vi "main.vi"() -> ()   [LabVIEW 2023]
uses:
  Lens Driver (20.06.2016)/03 Type Def & Global/Calibration.ctl
  <vilib>/Instr/_visa.llb/VISA Configure Serial Port (Instr).vi
panel:
  in  "Slide":dbl(slide) scale=0.0..10.0
  out "TA (°C)":dbl
  in  "Read Temperature":bool caption="Send Command"
  out "Command to Port":string
  in  "Current Ch A (mA)":dbl
  out "Data":string
  out "OK":bool
  out "Calibration 2":T1 {"Max Current A" format="%#_g mA"; "Max Current B" format="%#_g mA"; "UCL A" format="%#_g mA"; "LCL A" format="%#_g mA"; "UCL B" format="%#_g mA"; "LCL B" format="%#_g mA"}
  out "VISA resource name out":string
  in  "stop":bool
  in  "Send command":bool caption="Send Command"
  out "ID":u16
  out "error out":errorcluster
  in  "Calibration":T1={"Max Current A"=293.0, "Max Current B"=293.0, "UCL A"=300.0, "UCL B"=300.0, "LCL A"=0.0, "LCL B"=0.0} {"Max Current A" format="%#_g mA"; "Max Current B" format="%#_g mA"; "UCL A" format="%#_g mA"; "LCL A" format="%#_g mA"; "UCL B" format="%#_g mA"; "LCL B" format="%#_g mA"}
  in  "error in (no error)":errorcluster
  in  "VISA resource name":string="COM5"
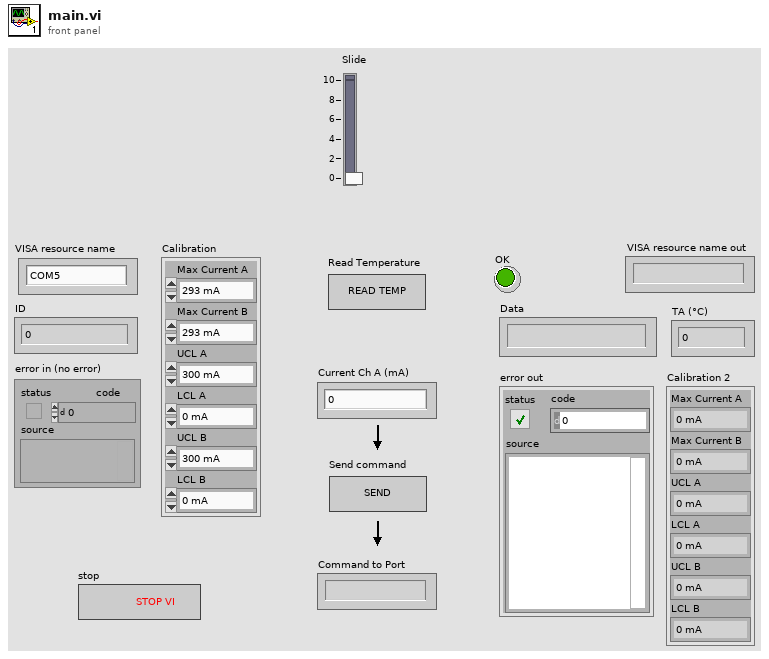
[diagram p1: front panel]
types:
  T1 = typedef "Calibration.ctl" = cluster{"Max Current A":dbl, "Max Current B":dbl, "UCL A":dbl, "UCL B":dbl, "LCL A":dbl, "LCL B":dbl}
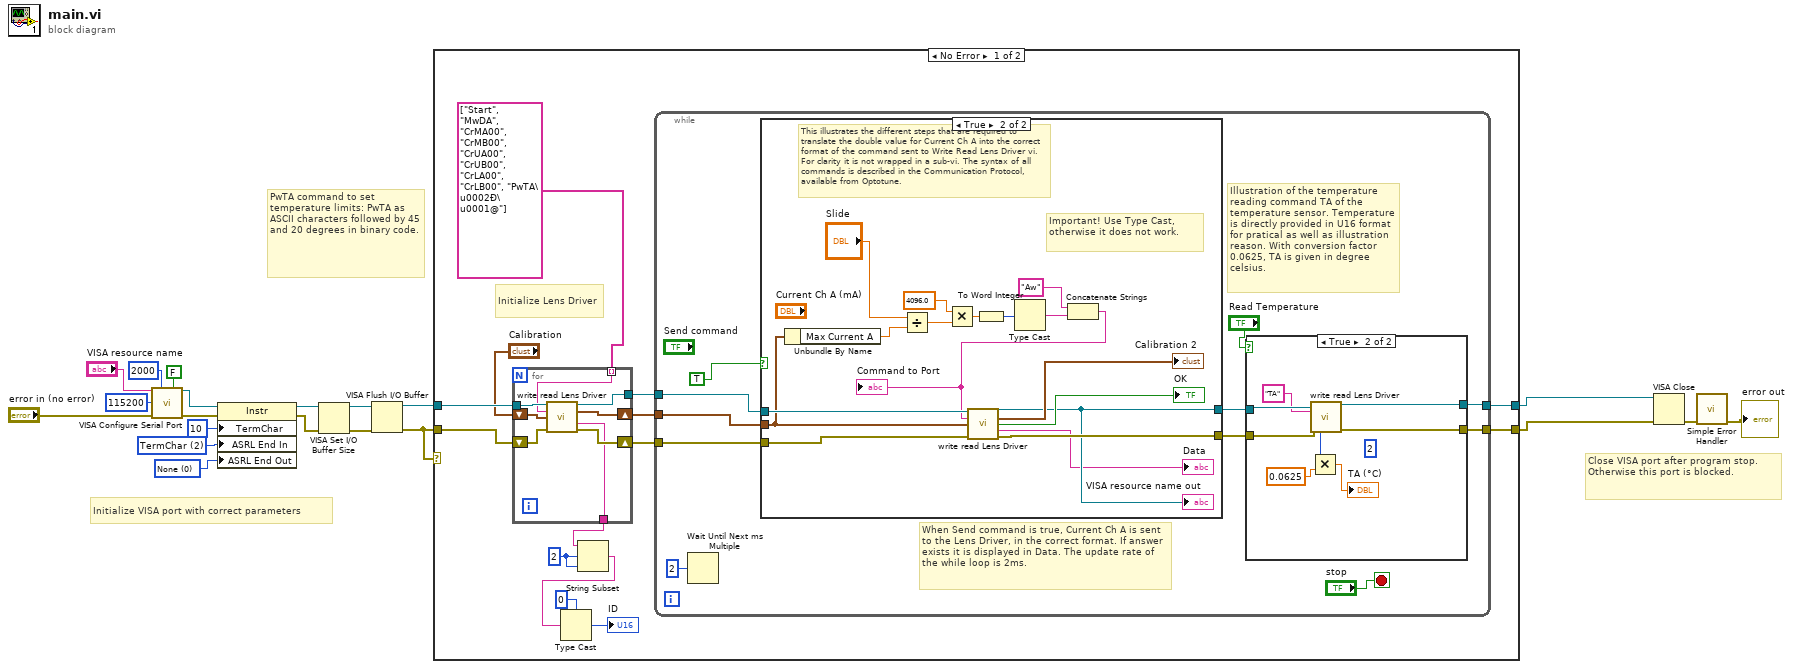
[diagram p0: block diagram]
diagram:
  w11 = u16 0 items=["None", "Last Bit", "TermChar", "Break"] ("Serial Settings:End Mode for Writes")
  w12 = u16 2 items=["None", "Last Bit", "TermChar"] ("Serial Settings:End Mode for Reads")
  # "PwTA command to set temperature limits: PwTA as ASCII characters followed by 45 and 20 degrees in binary code."
  # "Close VISA port after program stop. Otherwise this port is blocked."
  # "Initialize VISA port with correct parameters"
  n1 = call-poly "VISA Configure Serial Port"("VISA resource name"="VISA resource name", "timeout (10sec)"=u32 2000, "Enable Termination\nChar (T)"=FALSE ("Enable Termination\nChar (T)"), "baud rate (9600)"=u32 115200, "error in (no error)"="error in (no error)") -> ("VISA resource name out"=w16:refnum<visa-resource-name>, "error out"=w14:errorcluster)  [unwired: 9 in]
  n2 = property class="Instr"(reference=w16, error in=w14, "TermChar"=u8 10 ("Message Based Settings:Termination Character"), "ASRL End In"=w12, "ASRL End Out"=w11) -> (reference out=w15:refnum<visa-resource-name>, error out=w13:errorcluster)
  n3 = VISA Set I/O Buffer Size(VISA resource name=w15, error in (no error)=w13) -> (VISA resource name out=w8:refnum<visa-resource-name>, error out=w7:errorcluster)  [unwired: 2 in]
  n4 = VISA Flush I/O Buffer(VISA resource name=w8, error in (no error)=w7) -> (VISA resource name out=w6:refnum<visa-resource-name>, error out=w1:errorcluster)  [unwired: 1 in]
  n5 = case shown="No Error" w1 {
    tunnel: w1 -> [w34 w83]
    tunnel: w6 -> [w33 w84]
    tunnel: [w32 w83] -> w4
    tunnel: [w31 w84] -> w2
    frame No Error {
      w29 = 2 ("length (rest)")
      # "Initialize Lens Driver"
      n6 = for {
        tunnel: w33 -> [w81]
        tunnel: [w78] -> w23
        tunnel: string[] ["Start", "MwDA", "CrMA00", "CrMB00", "CrUA00", "CrUB00", "CrLA00", "CrLB00", "PwTA\u0002Ð\u0001@"] -> [w76] mode=indexing
        tunnel: [w75] -> w22
        shift-right: [w79] -> w24
        shift-left: "Calibration" -> [w80]
        shift-right: [w77] -> w25
        shift-left: w34 -> [w82]
        n7 = call "write read Lens Driver.vi"("VISA resource name"=w81, "command"=w76, "Calibration"=w80, "error in (no error)"=w82) -> ("VISA resource name out"=w78:refnum<visa-resource-name>, "Calibration 2"=w79:T1, "Data"=w75:string, "error out"=w77:errorcluster)  [unwired: 4 in, 4 out]
      }
      n8 = String Subset(string=w22, offset (0)=w29, length (rest)=w29) -> (substring=w27:string)
      n9 = Type Cast(type=u16 0 ("length (rest)"), x=w27) -> (*(type *) &x=→"ID":u16)
      n10 = while {
        tunnel: [w39] -> w32
        tunnel: [w40] -> w31
        tunnel: w25 -> [w45]
        tunnel: w24 -> [w44]
        tunnel: w23 -> [w43]
        stop <- "stop" stop-if-true
        # "Illustration of the temperature reading command TA of the temperature sensor. Temperature is directly provided in U16 format for pratical as well as illustration reason. With conversion factor 0.0625, TA is given in degree celsius."
        # "When Send command is true, Current Ch A is sent to the Lens Driver, in the correct format. If answer exists it is displayed in Data. The update rate of the while loop is 2ms."
        n11 = Wait Until Next ms Multiple(millisecond multiple=u32 2) -> ()  [unwired: 1 out]
        n12 = case shown="True" TRUE {
          tunnel: [w57 w74] -> w37
          tunnel: w45 -> [w57 w73]
          tunnel: w44 -> [_ w67]
          tunnel: w43 -> [w56 w72]
          tunnel: [w56 w69] -> w38
          frame False {
          }
          frame True {
            # "This illustrates the different steps that are required to translate the double value for Current Ch A into the correct format of the command sent to Write Read Lens Driver vi.  For clarity it is not wrapped in a sub-vi. The syntax of all commands is described in the Communication Protocol, available from Optotune."
            # "Important! Use Type Cast, otherwise it does not work."
            n13 = Unbundle By Name(w67) -> ("Max Current A"=w59:dbl)
            n14 = Divide(x="Slide", y=w59) -> (x/y=w66:dbl)
            n15 = Multiply(x=4096.0, y=w66) -> (x*y=w64:dbl)
            n16 = To Word Integer(number=w64) -> (16bit integer=w63:i16)
            n17 = Type Cast(x=w63) -> (*(type *) &x=w62:string)  [unwired: 1 in]
            n18 = Concatenate Strings("Aw", w62) -> (w60:string)
            "Command to Port" <- w60
            n19 = call "write read Lens Driver.vi"("VISA resource name"=w72, "command"=w60, "Calibration"=w67, "error in (no error)"=w73) -> ("VISA resource name out"=w69:refnum<visa-resource-name>, "Calibration 2"=→"Calibration 2":T1, "OK"=→"OK":bool, "Data"=→"Data":string, "error out"=w74:errorcluster)  [unwired: 4 in, 3 out]
            "VISA resource name out" <- w69
          }
        }
        n20 = case shown="True" "Read Temperature" {
          tunnel: [w47 w55] -> w40
          tunnel: [w46 w54] -> w39
          tunnel: w38 -> [w47 w53]
          tunnel: w37 -> [w46 w52]
          frame False {
          }
          frame True {
            (unwired) 2 ("length (rest)")
            n21 = call "write read Lens Driver.vi"("VISA resource name"=w53, "command"="TA", "error in (no error)"=w52) -> ("VISA resource name out"=w55:refnum<visa-resource-name>, "TA"=w49:u16, "error out"=w54:errorcluster)  [unwired: 5 in, 5 out]
            n22 = Multiply(x=w49, y=0.0625) -> (x*y=→"TA (°C)":dbl)
          }
        }
      }
    }
    frame Error {
    }
  }
  n23 = VISA Close(VISA resource name=w2, error in (no error)=w4) -> (error out=w5:errorcluster)
  n24 = call <vilib>:"Simple Error Handler.vi"("error in (no error)"=w5) -> ("error out"=→"error out":errorcluster)  [unwired: 4 in, 4 out]
